vi "GET Actuation Direction.vi"() -> (0 "Actuation Mode":T1)   [LabVIEW 2013]
uses:
  Actuation Mode.ctl
  Action.ctl
  Experimental Parameters FGV Selector.ctl
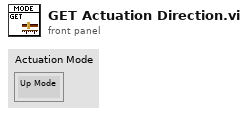
[diagram p1: front panel]
types:
  T1 = typedef "Actuation Mode.ctl" = enum16{"Up Mode", "Down Mode"}
  T2 = typedef "Experimental Parameters FGV Selector.ctl" = enum16{"Number of Samples", "Actuation Direction", "Ramp Rate"}
  T3 = typedef "Action.ctl" = enum16{"GET", "PUT", "DELETE"}
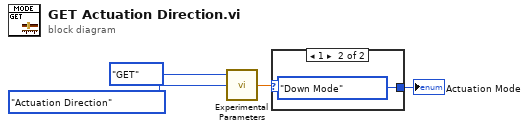
[diagram p0: block diagram]
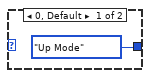
[diagram p2: hidden frame]
diagram:
  n1 = call "Experimental Parameters.vi"("Experimental Parameters FGV Selector"=Experimental_Parameters_FGV_Selector."Actuation Direction", "Action"=Action."GET") -> ("Output"=w4:dbl)  [unwired: 1 in]
  n2 = case shown="1" w4 {
    tunnel: [Actuation_Mode."Up Mode" ("Actuation Mode 2") Actuation_Mode."Down Mode" ("Actuation Mode 2")] -> w3
    frame 0, Default {
    }
    frame 1 {
    }
  }
  "Actuation Mode" <- w3
